vi "INTELLIFAUCET Core Start Stop.vi"(5 "Mode":T1=enum."Stop Flow", 6 "Debug":bool, 7 "mS wait":u32=500, 8 "error in (no error)":errorcluster, 10 "HEWH MW100 Channel Numbers":T2="011", 11 "VISA Refnum in":refnum<visa-resource-name>) -> (0 "error out":errorcluster, 3 "VISA Refnum out":refnum<visa-resource-name>)   [LabVIEW 2023]
uses:
  Type Definitions/HEWH Normally Open Valve Control.ctl
  MW100/Type Definitions/HEWH MW100 Channel Numbers.ctl
  Type Definitions/INTELLIFAUCET Set Mode.ctl
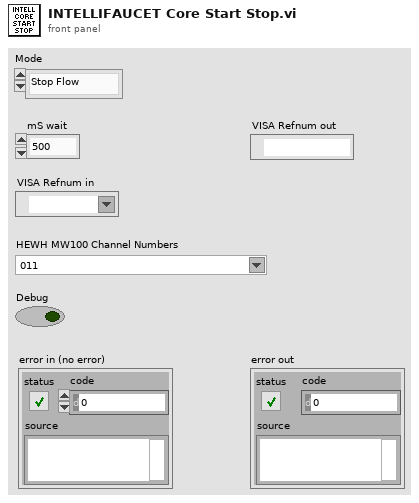
[diagram p1: front panel]
types:
  T1 = typedef "INTELLIFAUCET Set Mode.ctl" = enum16{"Adjust Temp", "Adjust Flow", "Start Flow", "Stop Flow", "Hold Start", "Hold Stop", "Release Start", "Release Stop", "Temp/Flow Relay", "Adjust Prop Valve"}
  T2 = typedef "HEWH MW100 Channel Numbers.ctl" = string
  T3 = typedef "HEWH Normally Open Valve Control.ctl" = string
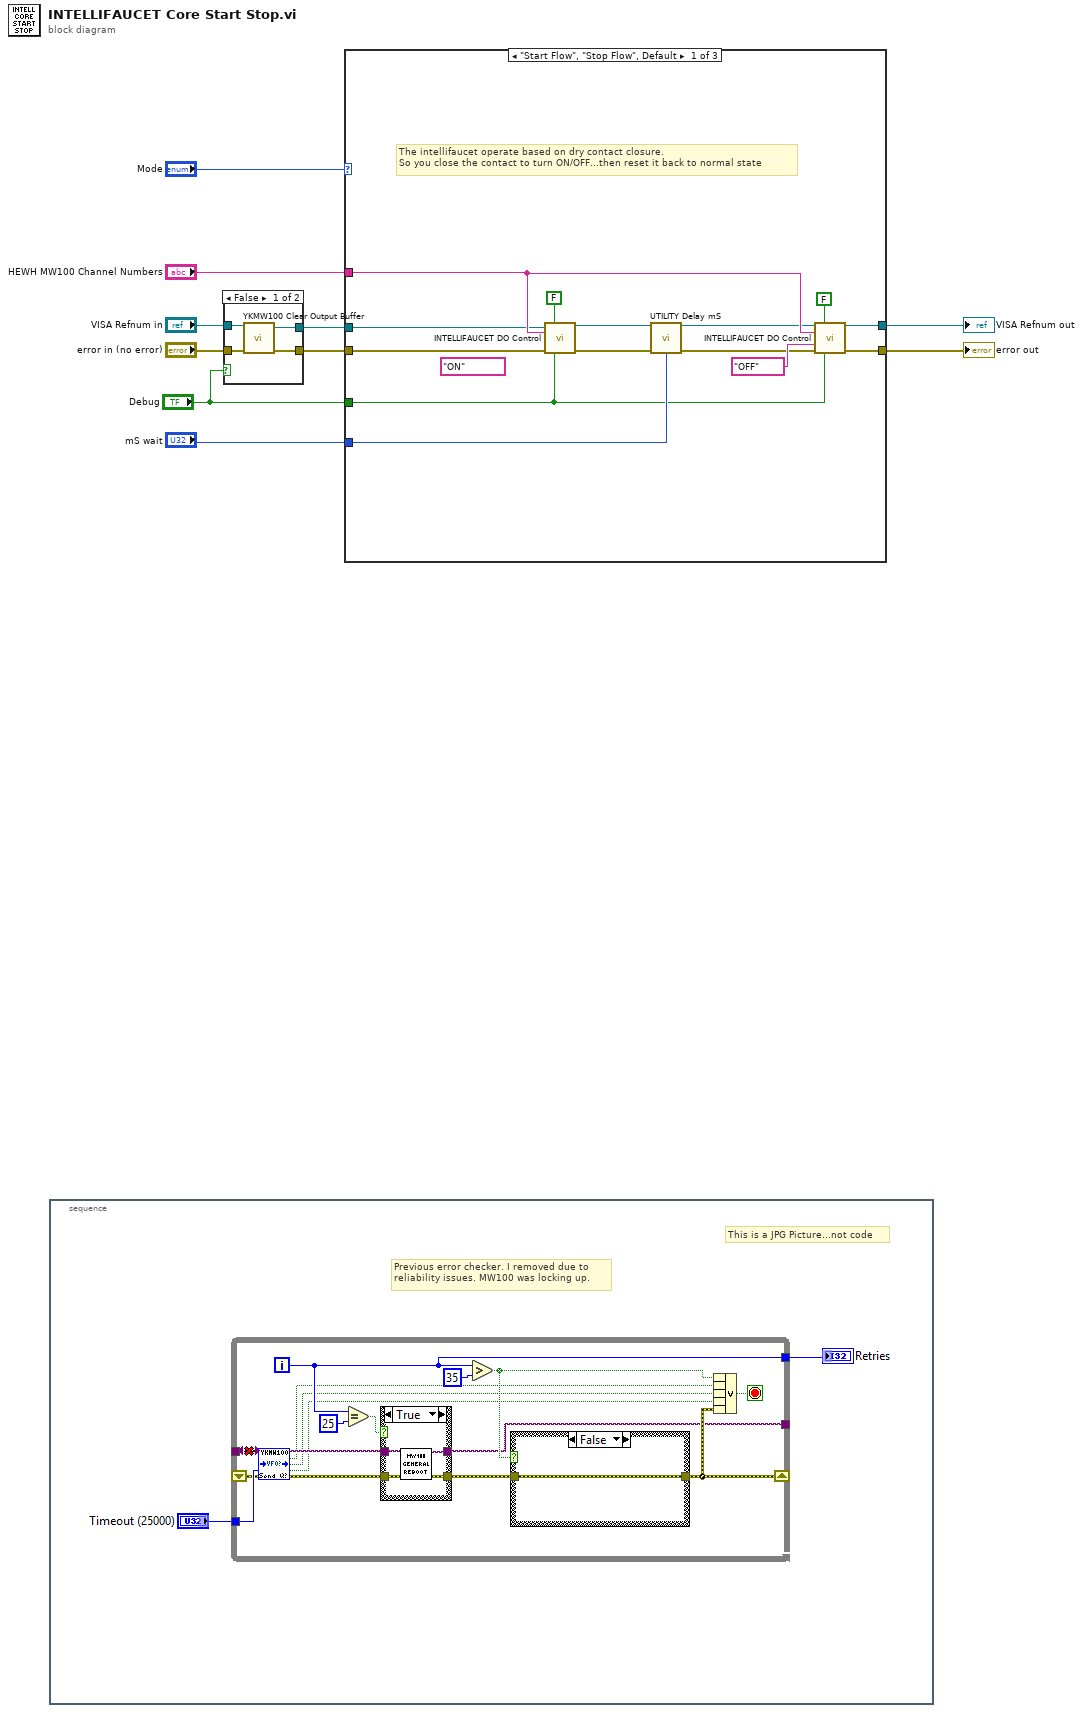
[diagram p0: block diagram]
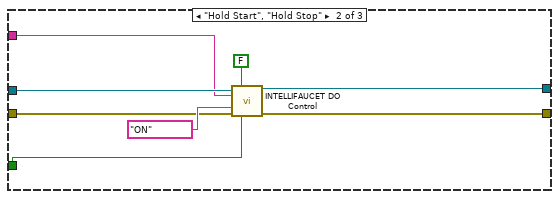
[diagram p3: hidden frame]
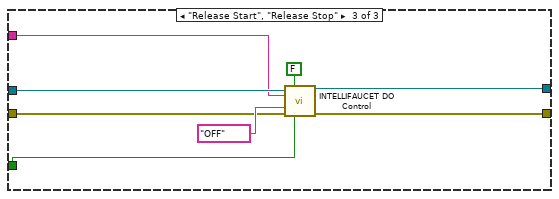
[diagram p4: hidden frame]
diagram:
  n1 = stacked-sequence {
    frame #0 {
      # "This is a JPG Picture...not code"
      # "Previous error checker. I removed due to \nreliability issues. MW100 was locking up."
    }
  }
  n2 = case shown="False" "Debug" {
    tunnel: "VISA Refnum in" -> [w14 w16]
    tunnel: "error in (no error)" -> [w13 w15]
    tunnel: [w12 w15] -> w5
    tunnel: [w11 w16] -> w4
    frame False {
      n3 = call "YKMW100 Clear Output Buffer.vi"("VISA session"=w14, "error in (no error)"=w13) -> ("dup VISA session"=w11:refnum<visa-resource-name>, "error out"=w12:errorcluster)  [unwired: 12 in]
    }
    frame True {
    }
  }
  n4 = case shown="\"Start Flow\", \"Stop Flow\", Default" "Mode" {
    tunnel: [w29 w31 w42] -> w10
    tunnel: [w28 w32 w41] -> w9
    tunnel: "HEWH MW100 Channel Numbers" -> [w27 w33 w39]
    tunnel: w5 -> [w26 w35 w43]
    tunnel: w4 -> [w25 w34 w40]
    tunnel: "mS wait" -> [w22 _ _]
    tunnel: "Debug" -> [w17 w30 w38]
    frame "Start Flow", "Stop Flow", Default {
      (unwired) T3 "ON" ("Normally Open Valve")
      # "The intellifaucet operate based on dry contact closure. \nSo you close the contact to turn ON/OFF...then reset it back to normal state"
      n5 = call "INTELLIFAUCET DO Control.vi"("VISA session"=w25, 1:FALSE ("Normally Closed Valve?"), "HEWH MW100 Channel Numbers"=w27, "Error In"=w26, 12:w17) -> ("dup VISA session"=w24:refnum<visa-resource-name>, "error out"=w21:errorcluster)  [unwired: 9 in]
      n6 = call "UTILITY Delay mS.vi"("Error In"=w21, "milliseconds to wait"=w22) -> ("Error Out"=w18:errorcluster)  [unwired: 13 in]
      n7 = call "INTELLIFAUCET DO Control.vi"("VISA session"=w24, 1:FALSE ("Normally Closed Valve?"), "HEWH MW100 Channel Numbers"=w27, 9:T3 "OFF" ("Normally Open Valve"), "Error In"=w18, 12:w17) -> ("dup VISA session"=w28:refnum<visa-resource-name>, "error out"=w29:errorcluster)  [unwired: 8 in]
    }
    frame "Hold Start", "Hold Stop" {
      n8 = call "INTELLIFAUCET DO Control.vi"("VISA session"=w34, 1:FALSE ("Normally Closed Valve?"), "HEWH MW100 Channel Numbers"=w33, 9:T3 "ON" ("Normally Open Valve"), "Error In"=w35, 12:w30) -> ("dup VISA session"=w32:refnum<visa-resource-name>, "error out"=w31:errorcluster)  [unwired: 8 in]
    }
    frame "Release Start", "Release Stop" {
      n9 = call "INTELLIFAUCET DO Control.vi"("VISA session"=w40, 1:FALSE ("Normally Closed Valve?"), "HEWH MW100 Channel Numbers"=w39, 9:T3 "OFF" ("Normally Open Valve"), "Error In"=w43, 12:w38) -> ("dup VISA session"=w41:refnum<visa-resource-name>, "error out"=w42:errorcluster)  [unwired: 8 in]
    }
  }
  "error out" <- w10
  "VISA Refnum out" <- w9
